vi "GetFirstPaneOrigin__slk_mt.vi"(8 "error in (no error)":errorcluster, 11 "vi refnum in":refnum<vi>) -> (0 "error out":errorcluster, 3 "origin":T1)   [LabVIEW 2012, in "Lazyboots Menu Tool.lvlib"]
doc: "Returns the origin of first pane."
uses:
  Library/Lazyboots Menu Tool.lvlib
  <vilib>/Utility/miscctls.llb/LVPointTypeDef.ctl
panel:
  # "GetFirstPaneOrigin__slk_mt.vi\nReturns the origin of first pane.\n\nNOTICE -- YOU MUST LEAVE THIS NOTICE IN PLACE.\n\nCopyright (c) 2011, LIANG LIU Shawn.Liu.cn@gmail.com\nAll rights reserved.\n\nRedistribution and use in source and binary forms, with or without modification, are permitted provided that the following conditions are met:\n-Redistributions of source code must retain the above copyright notice, this list of conditions and the following disclaimer.\n-Redistributions in binary form must reproduce the above copyright notice, this list of conditions and the following disclaimer in the documentation and/or other materials provided with the distribution.\n-Neither the name of the eLp nor the names of its contributors may be used to endorse or promote products derived from this software without specific prior written permission.\n\nTHIS SOFTWARE IS PROVIDED BY THE COPYRIGHT HOLDERS AND CONTRIBUTORS \"AS IS\" AND ANY EXPRESS OR IMPLIED WARRANTIES, INCLUDING, BUT NOT LIMITED TO, THE IMPLIED WARRANTIES OF MERCHANTABILITY AND FITNESS FOR A PARTICULAR PURPOSE ARE DISCLAIMED. IN NO EVENT SHALL THE COPYRIGHT HOLDER OR CONTRIBUTORS BE LIABLE FOR ANY DIRECT, INDIRECT, INCIDENTAL, SPECIAL, EXEMPLARY, OR CONSEQUENTIAL DAMAGES (INCLUDING, BUT NOT LIMITED TO, PROCUREMENT OF SUBSTITUTE GOODS OR SERVICES; LOSS OF USE, DATA, OR PROFITS; OR BUSINESS INTERRUPTION) HOWEVER CAUSED AND ON ANY THEORY OF LIABILITY, WHETHER IN CONTRACT, STRICT LIABILITY, OR TORT (INCLUDING NEGLIGENCE OR OTHERWISE) ARISING IN ANY WAY OUT OF THE USE OF THIS SOFTWARE, EVEN IF ADVISED OF THE POSSIBILITY OF SUCH DAMAGE."
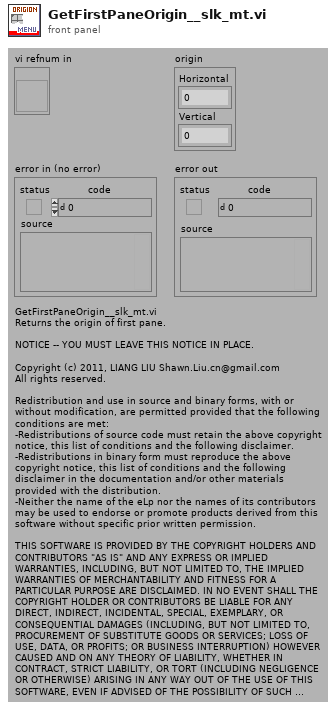
[diagram p1: front panel]
types:
  T1 = typedef "LVPointTypeDef.ctl" = cluster{"Horizontal":i16, "Vertical":i16}
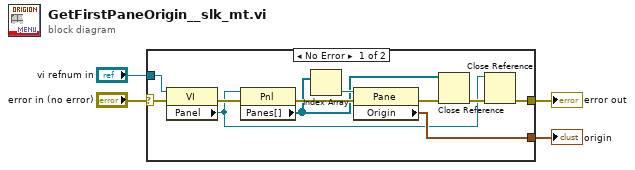
[diagram p0: block diagram]
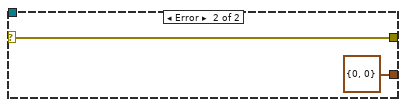
[diagram p2: hidden frame]
diagram:
  n1 = case shown="No Error" "error in (no error)" {
    selector: "error in (no error)" -> [w14 w17]
    tunnel: [w15 T1 {"Horizontal"=0, "Vertical"=0} ("Origin")] -> w4
    tunnel: [w13 w17] -> w2
    tunnel: "vi refnum in" -> [w5 _]
    frame No Error {
      n2 = property class="VI"(reference=w5, error in=w14) -> (error out=w12:errorcluster, "Panel"=w6:refnum<vi>)  [unwired: 1 out]
      n3 = property class="Pnl"(reference=w6, error in=w12) -> (error out=w10:errorcluster, "Panes[]"=w7:refnum<vi>[])  [unwired: 1 out]
      n4 = Index Array(array=w7) -> (element=w11:refnum<vi>)  [unwired: 1 in]
      n5 = property class="Pane"(reference=w11, error in=w10) -> (error out=w9:errorcluster, "Origin"=w15:T1)  [unwired: 1 out]
      n6 = Close Reference(reference=w7, error in (no error)=w9) -> (error out=w8:errorcluster)
      n7 = Close Reference(reference=w6, error in (no error)=w8) -> (error out=w13:errorcluster)
    }
    frame Error {
    }
  }
  "origin" <- w4
  "error out" <- w2
